vi "CDMA_Rx_Main.vi"() -> ()   [LabVIEW 2015]
uses:
  LabviewSubVI/RFConfig/StudentMsg.ctl
  LabviewSubVI/RFConfig/RF_Config.ctl
panel:
  in  "信道类型":enum16{"虚拟仿真", "真实系统"}(ring)
  in  "PC IP":string="192.168.1.215"
  in  "XSRP IP":string="192.168.1.145"
  out "导频信号星座图":cdb[](graph)
  out "接收端星座图":cdb[](graph)
  out "CRCFlag":u16 min=1 max=8
  out "主扰码号":u16=2 min=1 max=8
  out "扰码组号":u16=1 min=1 max=64
  in  "扩频码号":u16(ring)=1 items=["1"=1, "2"=2, "3"=3, "4"=4, "5"=5, "6"=6, "7"=7]
  in  "CRC 位数":u16(ring)=8 items=["0"=0, "8"=8, "12"=12, "16"=16, "24"=24]
  in  "?":T1={"发射频率"=2000000000, "发射衰减"=20, "接收频率"=2000000000, "接收增益"=0, "接收通道"=enum."RxCh1", "发射通道"=enum."TxCh1"} {"接收增益" max=40 format="%.0fdB"; "接收频率" min=70000000 max=6000000000 format="%.9pHz"; "发射衰减" max=90 format="%.0fdB"; "发射频率" min=70000000 max=6000000000 format="%.9pHz"}
  in  "扩频因子":u16(ring)=128 items=["8"=8, "16"=16, "32"=32, "64"=64, "128"=128]
  in  "编码方式":u16(ring)=1 items=["不编码", "1/2卷积码", "1/3卷积码"]
  out "时隙同步相关峰":dbl[](graph)
  out "接收字符信息":string
  out "实验学生信息":T2={"姓名"="XXX\n", "学号"="XXX", "班级"="XXX", "学校"="XXX"}
  # "基于XSRP软件无线电平台的CDMA通信系统接收机设计"
  # "实验参数设置"
  # "实验学生信息"
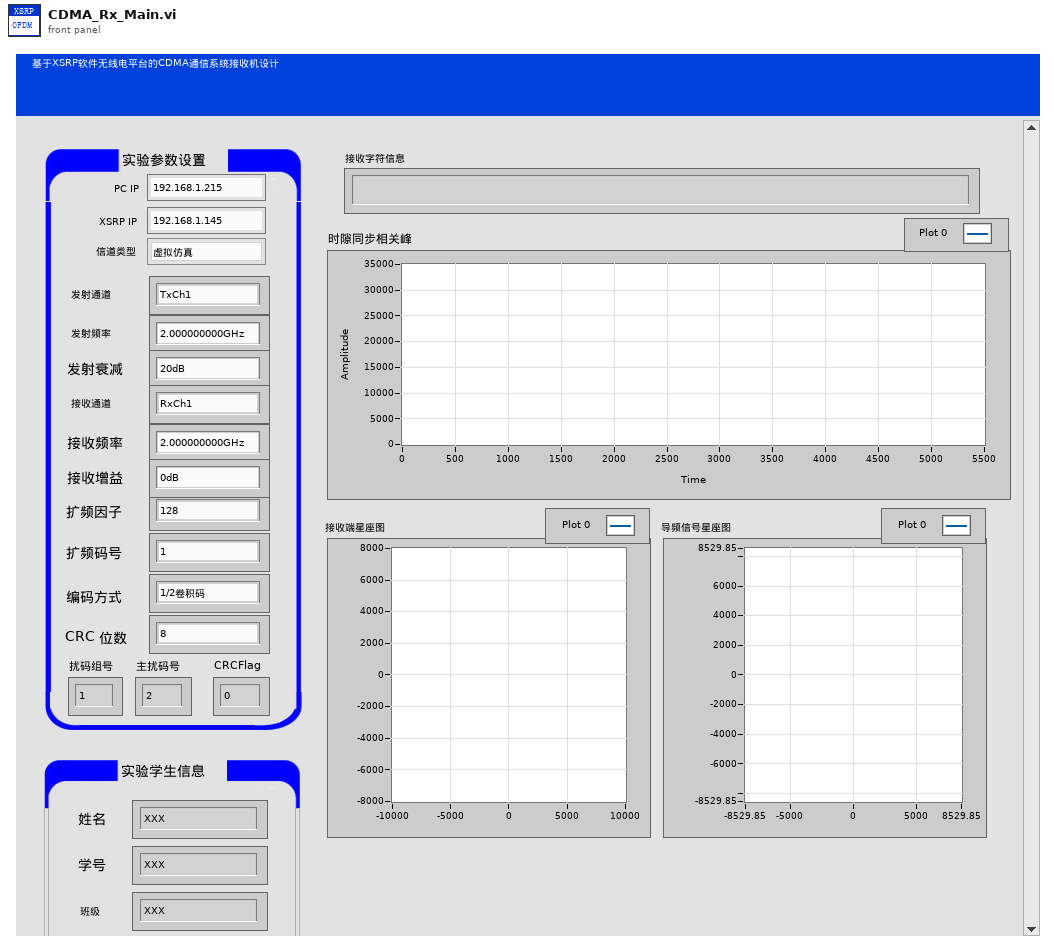
[diagram p1: front panel]
types:
  T1 = typedef "RF_Config.ctl" = cluster{"发射频率":u64, "发射衰减":u8, "接收频率":u64, "接收增益":u8, "接收通道":enum16{"RxCh1", "RxCh2"}, "发射通道":enum16{"TxCh1", "TxCh2"}}
  T2 = typedef "StudentMsg.ctl" = cluster{"姓名":string, "学号":string, "班级":string, "学校":string}
  T3 = cluster{"接收通道":enum16{"RxCh1", "RxCh2"}, "接收频率":u32, "接收增益":u8}
  T4 = cluster{"发射通道":enum16{"TxCh1", "TxCh2"}, "发射频率":u32, "发射衰减":u8}
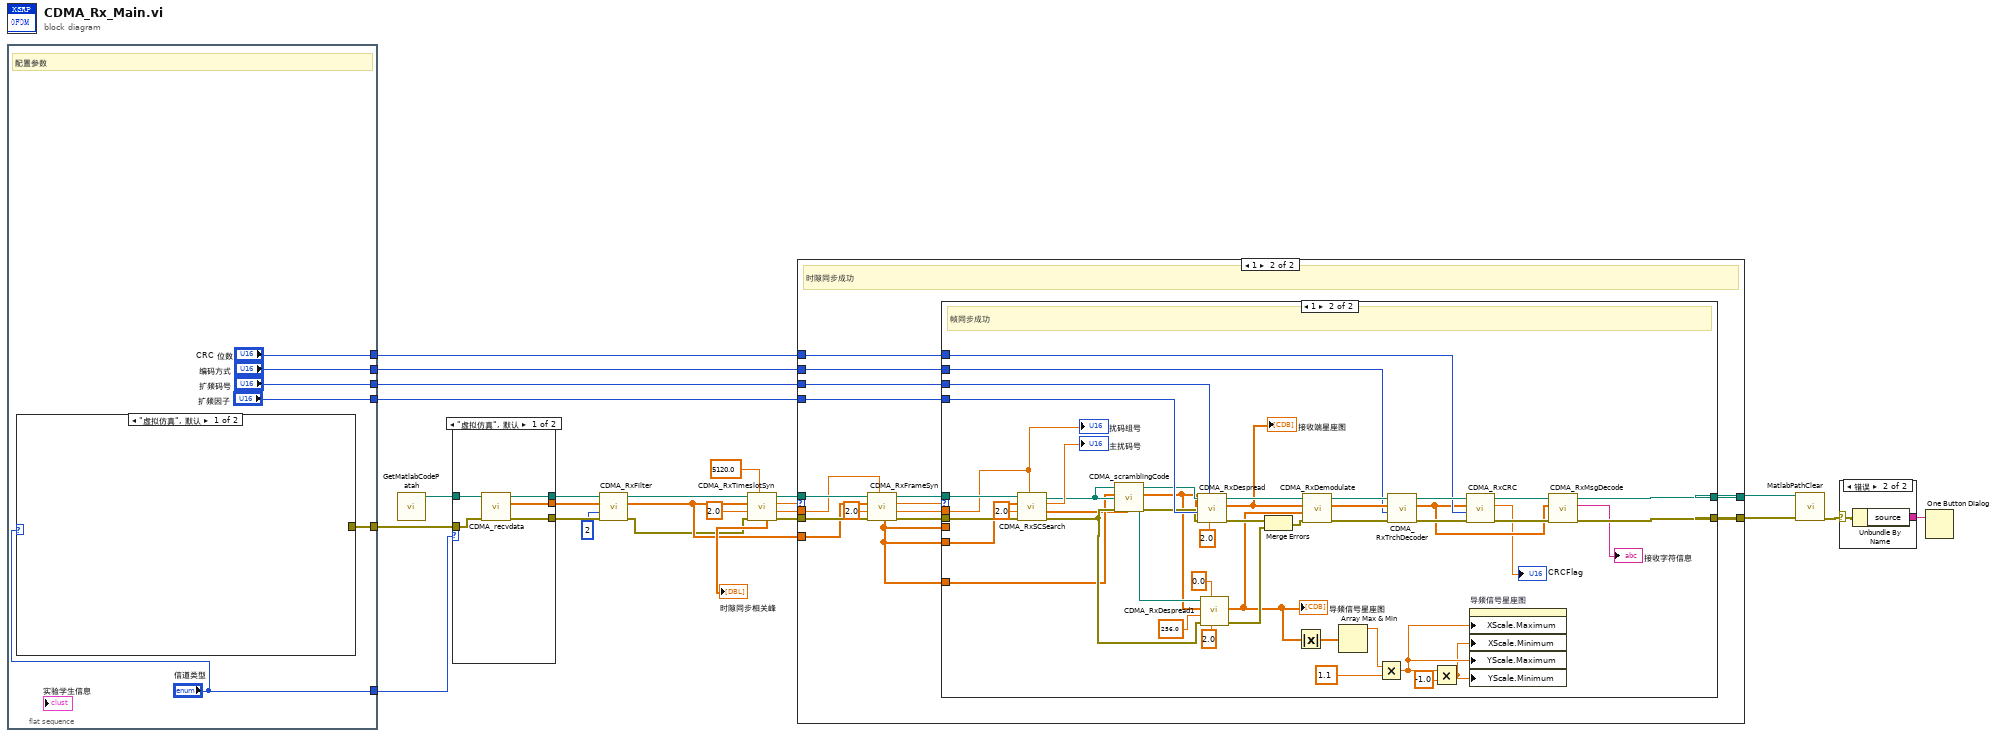
[diagram p0: block diagram]
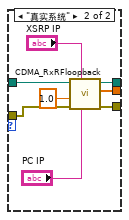
[diagram p2: hidden frame]
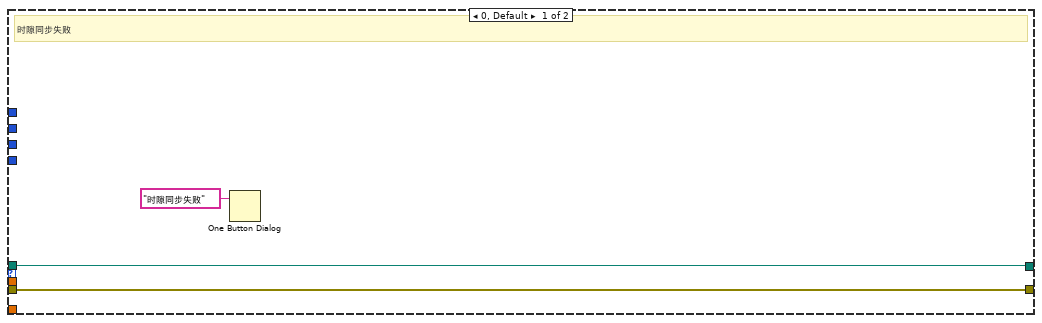
[diagram p3: hidden frame]
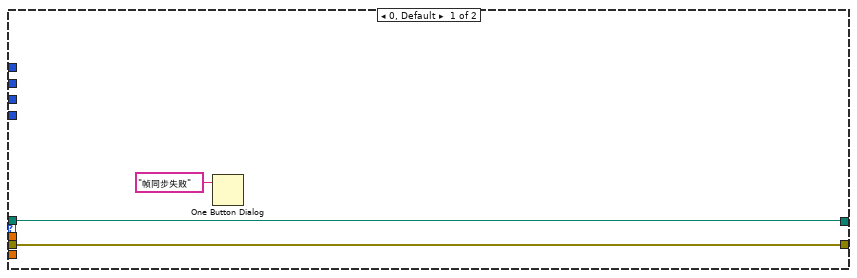
[diagram p4: hidden frame]
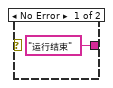
[diagram p5: hidden frame]
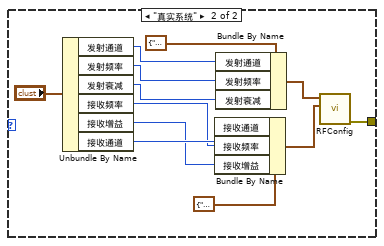
[diagram p6: hidden frame]
diagram:
  n1 = flat-sequence {
    tunnel: ["编码方式"] -> w13
    tunnel: ["扩频因子"] -> w15
    tunnel: [w29] -> w22
    tunnel: ["CRC 位数"] -> w10
    tunnel: ["扩频码号"] -> w14
    tunnel: ["信道类型"] -> w8
    frame #0 {
      # "配置参数"
      n2 = case shown="\"虚拟仿真\", 默认" "信道类型" {
        tunnel: [_ w32] -> w29
        frame "虚拟仿真", Default {
        }
        frame "真实系统" {
          n3 = Unbundle By Name("?") -> ("发射通道"=w40:enum16{"TxCh1", "TxCh2"}, "发射频率"=w39:u64, "发射衰减"=w38:u8, "接收频率"=w34:u64, "接收增益"=w35:u8, "接收通道"=w36:enum16{"RxCh1", "RxCh2"})
          n4 = Bundle By Name(cluster=T3 {"接收通道"=enum."RxCh1", "接收频率"=0, "接收增益"=0} ("接收参数设置"), "接收通道"=w36, "接收频率"=w34, "接收增益"=w35) -> (w33:T3)
          n5 = Bundle By Name(cluster=T4 {"发射通道"=enum."TxCh1", "发射频率"=0, "发射衰减"=0} ("发射参数设置"), "发射通道"=w40, "发射频率"=w39, "发射衰减"=w38) -> (w42:T4)
          n6 = call "RFConfig.vi"("接收参数设置"=w33, "发射参数设置"=w42) -> ("error out"=w32:errorcluster)  [unwired: 9 in]
        }
      }
    }
  }
  n7 = call "GetMatlabCodePatah.vi"() -> ("MatlabCodePath"=w23:path)  [unwired: 11 in]
  n8 = case shown="\"虚拟仿真\", 默认" w8 {
    tunnel: w23 -> [w48 w56]
    tunnel: w22 -> [w44 w55]
    tunnel: [w47 w53] -> w7
    tunnel: [w45 w52] -> w3
    tunnel: [w46 w51] -> w4
    frame "虚拟仿真", Default {
      n9 = call "CDMA_recvdata.vi"("error in (no error)"=w44, "Path"=w48) -> ("error out"=w45:errorcluster, "rx_data"=w46:cdb[], "Path Out"=w47:path)  [unwired: 7 in]
    }
    frame "真实系统" {
      n10 = call "CDMA_RxRFloopback.vi"("pcip"="PC IP", "xsrpip"="XSRP IP", "error in (no error)"=w55, "system_type"=1.0, "Path In"=w56) -> ("error out"=w52:errorcluster, "rxData"=w51:cdb[], "Path Out"=w53:path)  [unwired: 4 in]
    }
  }
  n11 = call "CDMA_RxFilter.vi"("error in (no error)"=w3, "sampleRate"=2, "rx_data"=w4, "Path"=w7) -> ("error out"=w2:errorcluster, "rxData"=w5:cdb[], "Path Out"=w6:path)  [unwired: 5 in]
  n12 = call "CDMA_RxTimeslotSyn.vi"("corr_length"=5120.0, "error in (no error)"=w2, "sampleRate"=2.0, "rx_data"=w5, "Path In"=w6) -> ("error out"=w16:errorcluster, "timeslot_star"=w17:dbl, "searchFlag"=w19:dbl, "Path Out"=w18:path, "PscCorr"=→"时隙同步相关峰":dbl[])  [unwired: 2 in]
  n13 = case shown="1" w19 {
    tunnel: w18 -> [w58 w75]
    tunnel: w17 -> [_ w68]
    tunnel: w16 -> [w57 w74]
    tunnel: w5 -> [_ w67]
    tunnel: w15 -> [_ w66]
    tunnel: w14 -> [_ w65]
    tunnel: w13 -> [_ w64]
    tunnel: [w58 w63] -> w12
    tunnel: [w57 w62] -> w11
    tunnel: w10 -> [_ w61]
    frame 0, Default {
      # "时隙同步失败"
      n14 = One Button Dialog(message="时隙同步失败") -> ()  [unwired: 1 in, 1 out]
    }
    frame 1 {
      # "时隙同步成功"
      n15 = call "CDMA_RxFrameSyn.vi"("timeslot_star"=w68, "error in (no error)"=w74, "sampleRate"=2.0, "rx_data"=w67, "Path In"=w75) -> ("error out"=w71:errorcluster, "scrambleGroupNo"=w69:dbl, "searchFlag1"=w70:dbl, "Path Out"=w72:path, "rx_data1"=w60:cdb[])  [unwired: 1 in, 1 out]
      n16 = case shown="1" w70 {
        tunnel: w72 -> [w77 w123]
        tunnel: w60 -> [_ w82]
        tunnel: w71 -> [w76 w122]
        tunnel: w69 -> [_ w100]
        tunnel: w66 -> [_ w118]
        tunnel: w65 -> [_ w117]
        tunnel: w64 -> [_ w110]
        tunnel: [w76 w109] -> w62
        tunnel: [w77 w107] -> w63
        tunnel: w61 -> [_ w102]
        tunnel: w60 -> [_ _]
        tunnel: w60 -> [_ w81]
        frame 0, Default {
          n17 = One Button Dialog(message="帧同步失败") -> ()  [unwired: 1 in, 1 out]
        }
        frame 1 {
          # "帧同步成功"
          n18 = call "CDMA_RxSCSearch.vi"("scrambleGroupNo"=w100, "error in (no error)"=w122, "sampleRate"=2.0, "rx_data1"=w82, "Path In"=w123) -> ("error out"=w84:errorcluster, "scramblingCode"=w80:cdb[], "scrambleNo"=→"主扰码号":dbl, "Path Out"=w86:path)  [unwired: 3 in]
          n19 = call "CDMA_scramblingCode.vi"("scramblingCode"=w80, "error in (no error)"=w84, "inputdata"=w81, "Path In"=w86) -> ("error out"=w83:errorcluster, "outdata"=w79:cdb[], "Path Out"=w85:path)  [unwired: 5 in]
          n20 = call "CDMA_RxDespread.vi"("sampleRate"=2.0, "ch_code_rx"=w117, "error in (no error)"=w83, "ch_sf_rx"=w118, "rx_data1"=w79, "Path In"=w85) -> ("error out"=w98:errorcluster, "pichData"=w94:cdb[], "Path Out"=w116:path)  [unwired: 3 in]
          "接收端星座图" <- w94
          n21 = call "CDMA_RxDespread1.vi"("sampleRate"=2.0, "ch_code_rx"=0.0, "error in (no error)"=w84, "ch_sf_rx"=256.0, "rx_data1"=w79, "Path In"=w86) -> ("error out"=w97:errorcluster, "pichData"=w93:cdb[])  [unwired: 3 in, 1 out]
          "导频信号星座图" <- w93
          n22 = Merge Errors(w98, w97) -> (w96:errorcluster)
          n23 = Absolute Value(x=w93) -> (abs(x)=w91:dbl[])
          n24 = call "CDMA_RxDemodulate.vi"("error in (no error)"=w96, "pichData"=w93, "dpchData"=w94, "Path In"=w116) -> ("error out"=w111:errorcluster, "dpchBit"=w113:dbl[], "Path  Out"=w112:path)  [unwired: 4 in, 1 out]
          n25 = Array Max & Min(array=w91) -> (max value=w90:dbl)  [unwired: 3 out]
          n26 = Multiply(x=w90, y=1.1) -> (x*y=w89:dbl)
          n27 = call "CDMA_RxTrchDecoder.vi"("error in (no error)"=w111, "rx_coder_type"=w110, "dpchBit"=w113, "Path In"=w112) -> ("error out"=w105:errorcluster, "ch_decode_data"=w101:dbl[], "Path Out"=w106:path)  [unwired: 5 in]
          n28 = Multiply(x=w89, y=-1.0) -> (x*y=w87:dbl)
          n29 = call "CDMA_RxCRC.vi"("error in (no error)"=w105, "rx_crc_num"=w102, "ch_decode_data"=w101, "Path In"=w106) -> ("error out"=w104:errorcluster, "CRC_flag"=→"CRCFlag":dbl, "Path Out"=w103:path)  [unwired: 5 in]
          n30 = property on="导频信号星座图" class="XYGraph (严格)"("XScale.Maximum"=w89, "XScale.Minimum"=w87, "YScale.Maximum"=w89, "YScale.Minimum"=w87) -> ()  [unwired: 2 in, 2 out]
          n31 = call "CDMA_RxMsgDecode.vi"("error in (no error)"=w104, "ch_decode_data"=w101, "Path In"=w103) -> ("error out"=w109:errorcluster, "char_msg"=→"接收字符信息":string, "Path  Out"=w107:path)  [unwired: 6 in]
          "扰码组号" <- w100
        }
      }
    }
  }
  n32 = call "MatlabPathClear.vi"("error in"=w11, "Path"=w12) -> ("error out"=w24:errorcluster)  [unwired: 9 in]
  n33 = case shown="错误" w24 {
    selector: w24 -> [_ w125]
    tunnel: ["运行结束" ("source") w126] -> w25
    frame No Error {
    }
    frame Error {
      n34 = Unbundle By Name(w125) -> ("source"=w126:string)
    }
  }
  n35 = One Button Dialog(message=w25) -> ()  [unwired: 1 in, 1 out]
